vi "VCI_Receive.vi"(6 "WaitTime":i16 caption="WaitTime(0ms)", 7 "Len":u32=2500 caption="Len(2500)", 8 "error in (no error)":errorcluster caption="错误输入（无错误）", 9 "CANIndex":u32, 10 "DevIndex":u32, 11 "DevType":T2=2 items=["USB-CAN"=2, "USB-CAN2"=3]) -> (0 "error out":errorcluster caption="错误输出", 3 "Recieve":T1[](array[typedef]))   [LabVIEW 2018, in "ControlCan.lvlib"]
uses:
  ControlCan.lvlib
  DevType.ctl
  VCI_CAN_OBJ.ctl
panel:
  in  "pBuff":u8[](array[numeric])
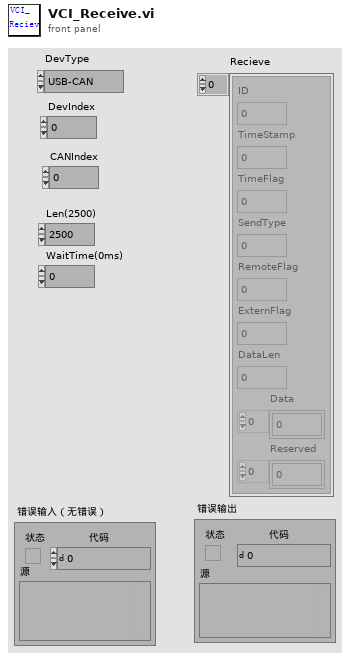
[diagram p1: front panel]
types:
  T1 = typedef "ControlCAN.lvlib/VCI_CAN_OBJ.ctl" = cluster{"ID":u32, "TimeStamp":u32, "TimeFlag":u8, "SendType":u8, "RemoteFlag":u8, "ExternFlag":u8, "DataLen":u8, "Data":u8[], "Reserved":u8[]}
  T2 = typedef "ControlCAN.lvlib/DevType.ctl" = u32
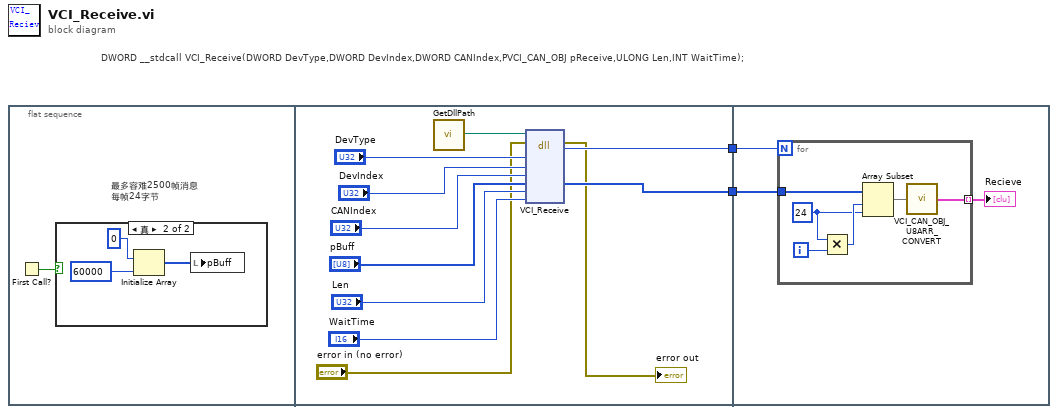
[diagram p0: block diagram]
diagram:
  # "DWORD __stdcall VCI_Receive(DWORD DevType,DWORD DevIndex,DWORD CANIndex,PVCI_CAN_OBJ pReceive,ULONG Len,INT WaitTime);"
  n1 = flat-sequence {
    tunnel: [w14] -> w2
    tunnel: [w13] -> w1
    tunnel: w2 -> [w20]
    tunnel: w1 -> [w19]
    frame #0 {
      # "最多容难2500帧消息\n每帧24字节"
      n2 = First Call?() -> (First Call?: T/F=w3:bool)
      n3 = case shown="真" w3 {
        frame False {
        }
        frame True {
          n4 = Initialize Array(u8 0, 60000 ("维数大小")) -> (w6:u8[])
          n5 = local write "pBuff"(w6) -> ()
        }
      }
    }
    frame #1 {
      n6 = call "GetDllPath.vi"() -> ("DllPath"=w7:path)  [unwired: 1 out]
      n7 = dll-call lib="?" fn="VCI_Receive"(path in=w7, error in="error in (no error)", "DevType"="DevType", "DevIndex"="DevIndex", "CANIndex"="CANIndex", "pReceive"="pBuff", "Len"="Len", "WaitTime"="WaitTime") -> (error out=→"error out":errorcluster, "ReturnVal"=w13:i32, "pReceive"=w14:u8[])  [unwired: 6 in, 1 out]
    }
    frame #2 {
      n8 = for {
        N: w19 -> [_]
        tunnel: w20 -> [w26]
        tunnel: [w21] -> w18 mode=indexing
        i -> [w25]
        w23 = 24 ("x")
        n9 = Multiply(x=w23, y=w25) -> (x*y=w24:i32)
        n10 = Array Subset(array=w26, index=w24, length=w23) -> (w22:u8[])
        n11 = call "VCI_CAN_OBJ_U8ARR_CONVERT.vi"("U8_Arr"=w22) -> ("VCI_CAN_OBJ"=w21:T1)
      }
      "Recieve" <- w18
    }
  }
